vi "EstimateHybridNodes.vi"(0 "X (in) [t0]":dbl, 1 "Hybrid Node Range Threshold (in)":dbl=8.0, 2 "Min Hybrid Node Observations":i32=10, 3 "Max Allowed Y Bias (in)":dbl=5.0 format="%#_13g", 5 "Y (in) [t0]":dbl, 9 "Hybrid Node Range (in) [t0]":dbl, 11 "TOF Valid [t0]":bool) -> (4 "Scored Hybrid Nodes":bool[](array[boolean]), 15 "Nearest Node":i32)   [LabVIEW 2020]
doc: "Keeps track of which hybrid nodes already have scored game pieces in them."
uses:
  <vilib>/Rock Robotics/WPI/DriverStation/WPI_DriverStationAllianceInfo.ctl
  6475e6d8-15a5-46b3-ab69-812e861f270c.vi
  GlobalDriverStationData.vi
  GlobalPoseAndTargeting.vi
  GlobalGripper.vi
  GlobalMiscellaneous.vi
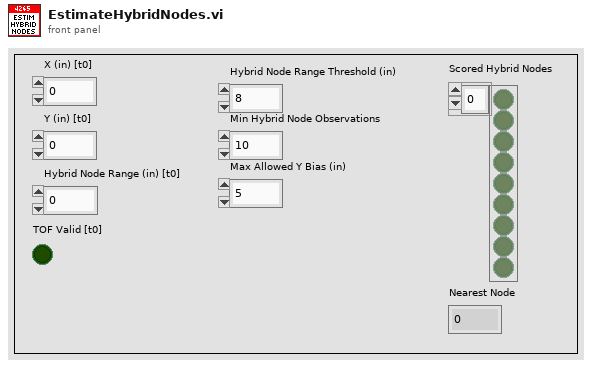
[diagram p1: front panel]
types:
  T1 = typedef "WPI_DriverStationAllianceInfo.ctl" = enum16{"Red", "Blue", "Invalid"}
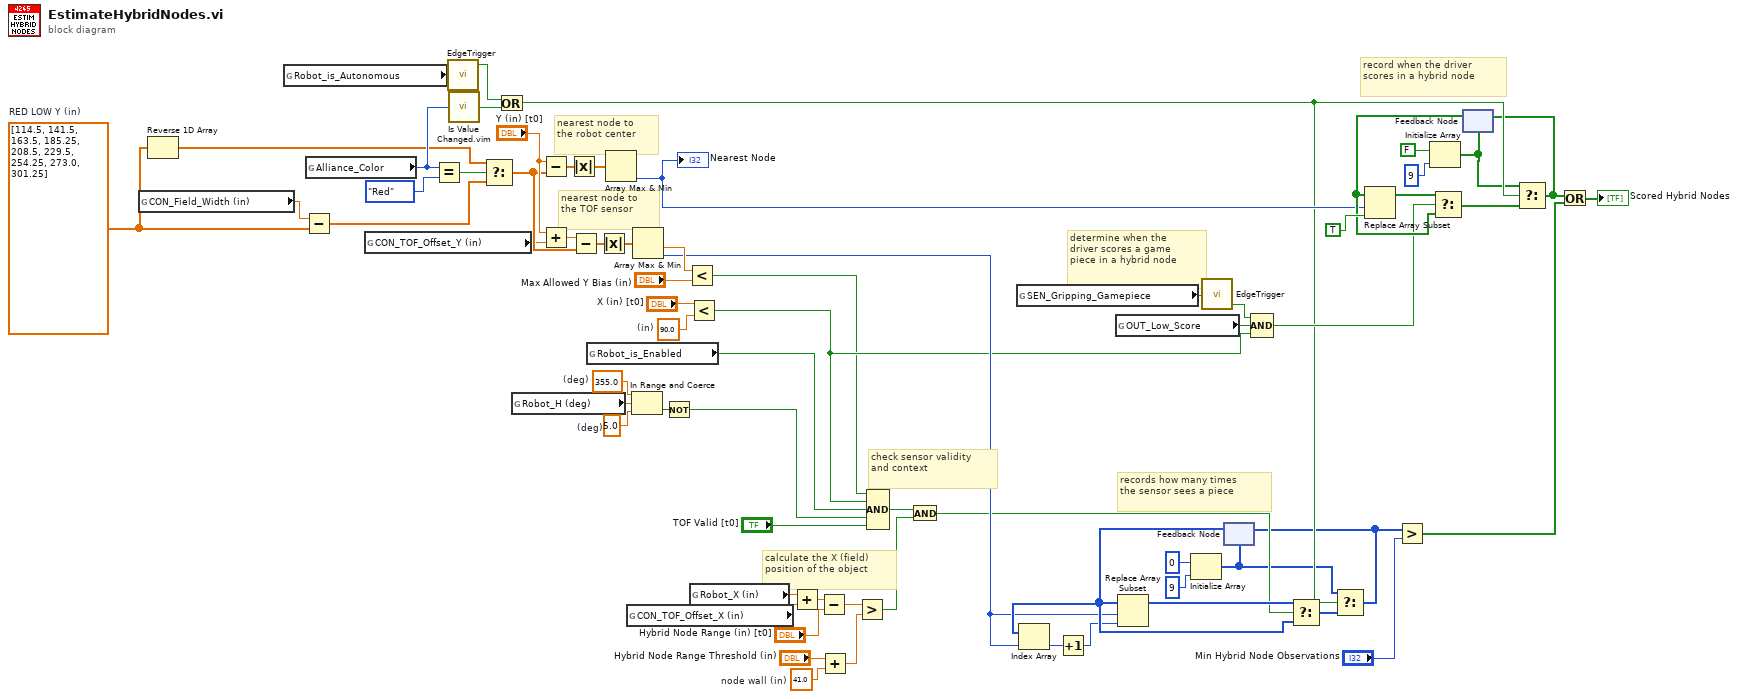
[diagram p0: block diagram]
diagram:
  w32 = 41.0  # node wall (in)
  w15 = 355.0  # (deg)
  w16 = 5.0  # (deg)
  w64 = 90.0  # (in)
  w66 = dbl[] [114.5, 141.5, 163.5, 185.25, 208.5, 229.5, 254.25, 273.0, 301.25]  # RED LOW Y (in)
  # "determine when the\ndriver scores a game\npiece in a hybrid node"
  # "calculate the X (field)\nposition of the object"
  # "check sensor validity\nand context"
  # "nearest node to\nthe TOF sensor"
  # "nearest node to\nthe robot center"
  # "records how many times\nthe sensor sees a piece"
  # "record when the driver\nscores in a hybrid node"
  n1 = global read "GlobalPoseAndTargeting.vi" "CON_Field_Width (in)"() -> (w68:dbl)
  n2 = Reverse 1D Array(array=w66) -> (reversed array=w56:dbl[])
  n3 = global read "GlobalDriverStationData.vi" "Robot_is_Autonomous"() -> (w47:bool)
  n4 = Subtract(x=w68, y=w66) -> (x-y=w57:dbl[])
  n5 = global read "GlobalDriverStationData.vi" "Alliance_Color"() -> (w63:T1)
  n6 = global read "GlobalMiscellaneous.vi" "CON_TOF_Offset_Y (in)"() -> (w13:dbl)
  n7 = Equal?(x=w63, y=WPI_DriverStationAllianceInfo."Red") -> (x = y?=w67:bool)
  n8 = call "EdgeTrigger.vi"("Input Signal"=w47) -> ("Rising Edge Trigger"=w45:bool)  [unwired: 2 out]
  n9 = call "Is Value Changed.vim"("value"=w63) -> ("changed or first call?"=w48:bool)
  n10 = Select(t=w56, s=w67, f=w57) -> (s? t:f=w22:dbl[])
  n11 = Or(x=w45, y=w48) -> (x .or. y?=w46:bool)
  n12 = global read "GlobalPoseAndTargeting.vi" "Robot_H (deg)"() -> (w54:dbl)
  n13 = Subtract(x="Y (in) [t0]", y=w22) -> (x-y=w27:dbl[])
  n14 = Add(x="Y (in) [t0]", y=w13) -> (x+y=w23:dbl)
  n15 = Absolute Value(x=w27) -> (abs(x)=w58:dbl[])
  n16 = Subtract(x=w23, y=w22) -> (x-y=w21:dbl[])
  n17 = global read "GlobalDriverStationData.vi" "Robot_is_Enabled"() -> (w36:bool)
  n18 = Absolute Value(x=w21) -> (abs(x)=w26:dbl[])
  n19 = Array Max & Min(array=w58) -> (min index (indices)=w50:i32)  [unwired: 3 out]
  "Nearest Node" <- w50
  n20 = global read "GlobalMiscellaneous.vi" "CON_TOF_Offset_X (in)"() -> (w14:dbl)
  n21 = In Range and Coerce(upper limit=w15, x=w54, lower limit=w16) -> (In Range?=w53:bool)  [unwired: 1 out]
  n22 = Array Max & Min(array=w26) -> (min value=w25:dbl, min index (indices)=w20:i32)  [unwired: 2 out]
  n23 = Not(x=w53) -> (.not. x?=w38:bool)
  n24 = Less?(x=w25, y="Max Allowed Y Bias (in)") -> (x < y?=w18:bool)
  n25 = Less?(x="X (in) [t0]", y=w64) -> (x < y?=w19:bool)
  n26 = global read "GlobalPoseAndTargeting.vi" "Robot_X (in)"() -> (w37:dbl)
  n27 = Add(x=w37, y=w14) -> (x+y=w35:dbl)
  n28 = Subtract(x=w35, y="Hybrid Node Range (in) [t0]") -> (x-y=w31:dbl)
  n29 = Add(x="Hybrid Node Range Threshold (in)", y=w32) -> (x+y=w30:dbl)
  n30 = Greater?(x=w31, y=w30) -> (0:w11:bool)
  n31 = Compound Arithmetic op=AND(w18, w19, w36, w38, "TOF Valid [t0]") -> (w12:bool)
  n32 = And(x=w12, y=w11) -> (x .and. y?=w10:bool)
  n33 = global read "GlobalGripper.vi" "SEN_Gripping_Gamepiece"() -> (w28:bool)
  n34 = global read "GlobalGripper.vi" "OUT_Low_Score"() -> (w29:bool)
  n35 = Initialize Array(0, 9 ("dimension size")) -> (w7:i32[])
  n36 = call "EdgeTrigger.vi"("Input Signal"=w28) -> ("Falling Edge Trigger"=w3:bool)  [unwired: 2 out]
  n37 = feedback #1(w7) -> (w49:i32[])
  n38 = Index Array(array=w49, index=w20) -> (element=w44:i32)
  n39 = Increment(x=w44) -> (x+1=w41:i32)
  n40 = Replace Array Subset(array=w49, new element=w41, index=w20) -> (w51:i32[])
  n41 = Compound Arithmetic op=AND(w3, w29, w19) -> (w55:bool)
  n42 = Select(t=w51, s=w10, f=w49) -> (s? t:f=w52:i32[])
  n43 = Select(t=w7, s=w46, f=w52) -> (s? t:f=w2:i32[])
  n44 = feedback-in #1(w2) -> ()
  n45 = Greater?(x=w2, y="Min Hybrid Node Observations") -> (0:w1:bool[])
  n46 = Initialize Array(FALSE, 9 ("dimension size")) -> (w4:bool[])
  n47 = feedback #2(w4) -> (w59:bool[])
  n48 = Replace Array Subset(array=w59, new element=TRUE ("new element/subarray"), index=w50) -> (w60:bool[])
  n49 = Select(t=w60, s=w55, f=w59) -> (s? t:f=w61:bool[])
  n50 = Select(t=w4, s=w46, f=w61) -> (s? t:f=w43:bool[])
  n51 = feedback-in #2(w43) -> ()
  n52 = Or(x=w43, y=w1) -> (x .or. y?=→"Scored Hybrid Nodes":bool[])
